vi "Get Version.vi"(6 "timeout (ms)":i32=5000, 8 "error in":errorcluster, 11 "gRPC ID":T2) -> (0 "error out":errorcluster, 2 "Version":T1, 3 "gRPC ID out":T2)   [LabVIEW 2021, in "CIFCoreWrapper.lvlib"]
uses:
  CIFCoreWrapper.lvlib
  CIFCorePlugin_client/CIFCorePlugin_client.lvlib
  Common/Typedef/Version.ctl
  Common/CIFCoreCommon.lvlib
  <vilib>/gRPC/LabVIEW gRPC Library/Shared/grpcId.ctl
  <vilib>/gRPC/LabVIEW gRPC Library/grpc-lvsupport-release.lvlib
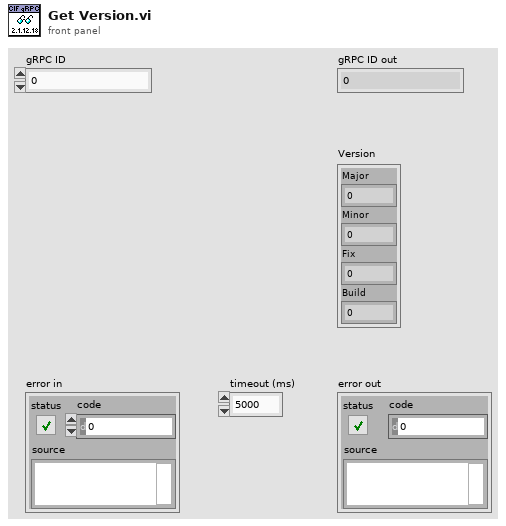
[diagram p1: front panel]
types:
  T1 = typedef "CIFCoreCommon.lvlib/Version.ctl" = cluster{"Major":i32, "Minor":i32, "Fix":i32, "Build":i32}
  T2 = typedef "grpc-lvsupport-release.lvlib/grpcId.ctl" = u64
  T3 = typedef "CIFCorePlugin_client.lvlib/cif_plugincore_GetVersionResponse.ctl" = cluster{"version":T4}
  T4 = typedef "CIFCorePlugin_client.lvlib/cif_common_Version.ctl" = cluster{"major":u32, "minor":u32, "fix":u32, "build":u32}
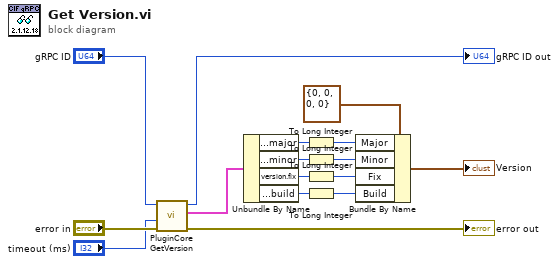
[diagram p0: block diagram]
diagram:
  n1 = call "PluginCore GetVersion.vi"("error in"="error in", "timeout (ms)"="timeout (ms)", "gRPC ID"="gRPC ID") -> ("error out"=→"error out":errorcluster, "Response Data"=w11:T3, "gRPC ID out"=→"gRPC ID out":T2)  [unwired: 6 in]
  n2 = Unbundle By Name(w11) -> ("version.major"=w9:u32, "version.minor"=w6:u32, "version.fix"=w7:u32, "version.build"=w8:u32)
  n3 = To Long Integer(number=w9) -> (32bit integer=w5:i32)
  n4 = To Long Integer(number=w6) -> (32bit integer=w4:i32)
  n5 = To Long Integer(number=w7) -> (32bit integer=w3:i32)
  n6 = To Long Integer(number=w8) -> (32bit integer=w2:i32)
  n7 = Bundle By Name(cluster=T1 {"Major"=0, "Minor"=0, "Fix"=0, "Build"=0} ("Version"), "Major"=w5, "Minor"=w4, "Fix"=w3, "Build"=w2) -> (→"Version":T1)
